vi "SetTOREG.vi"(8 "error in (no error)":errorcluster) -> (0 "error out":errorcluster)   [LabVIEW 2015, in "ESLSCDLL.lvlib"]
uses:
  ESLSCDLL.lvlib
  Globals.vi
panel:
  # "if (fkt==0)set to REG -> XCK\nif (fkt==1)set to REG -> OutTrig\nif (fkt==2)set to FFRead\nif (fkt==3)set to TrigIn\nif (fkt==4)set to EC\nif (fkt==5)set to DAT"
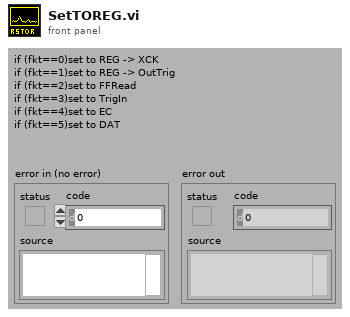
[diagram p1: front panel]
types:
  T1 = enum32{"XCK", "Reg/OutTrig", "VON", "DMA_Act", "ASLS", "STIMER", "BTIMER", "INTRSR", "S1", "S2", "BON", "MEASUREON", "SDAT", "BDAT", "SSHUT", "BSHUT", "IFC", "DO_CC_I", "EXPOSURE_WINDOW", "TO_CNT_OUT", "SECON", "I", "unused2", "unused3", "unused4", "unused5", "unused6", "unused7", "unused8", "ENFFR", "ENFFW", "ENFFWRPROT"}
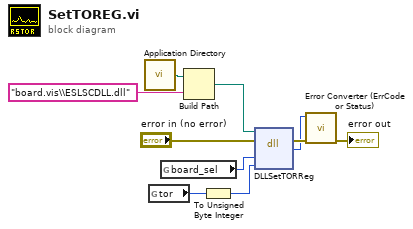
[diagram p0: block diagram]
diagram:
  n1 = call <vilib>:"Application Directory.vi"() -> ("Application Directory"=w4:path)
  n2 = global read "Globals.vi" "tor"() -> (w6:T1)
  n3 = global read "Globals.vi" "board_sel"() -> (w1:u32)
  n4 = Build Path(base path=w4, name or relative path="board.vis\\ESLSCDLL.dll") -> (appended path=w2:path)
  n5 = To Unsigned Byte Integer(number=w6) -> (unsigned 8bit integer=w5:u8)
  n6 = dll-call lib="C:/ENTW/PCIE/LV64/board.vis/ESLSCDLL.dll" fn="DLLSetTORReg" ("lwlscdll.dll:DLLRsTOREG")(path in=w2, error in="error in (no error)", "board_sel"=w1, "fkt"=w5) -> (error out=w8:errorcluster, "es_status_codes"=w7:i32)  [unwired: 3 in, 1 out]
  n7 = call "Error Converter (ErrCode or Status).vi"("error in (no error)"=w8, "error code"=w7) -> ("error out"=→"error out":errorcluster)  [unwired: 9 in]
